vi "SRV_Sensors Variant to Data.vi"(8 "error in (no error)":errorcluster, 10 "Data":variant, 11 "Command":string) -> (0 "error out":errorcluster, 2 "Data String":string)   [LabVIEW 2014]
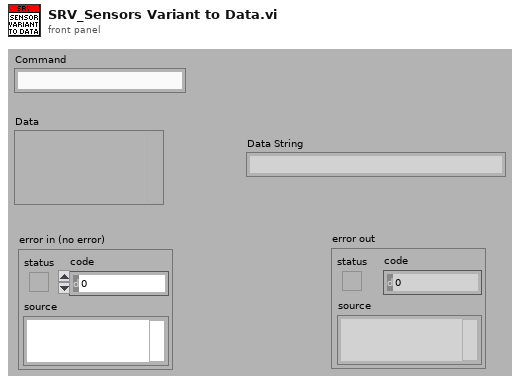
[diagram p1: front panel]
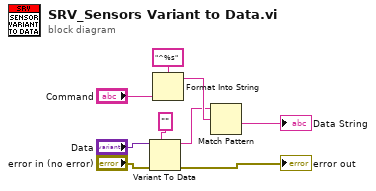
[diagram p0: block diagram]
diagram:
  n1 = Variant To Data(error in="error in (no error)", type="", Variant="Data") -> (data=w5:string, error out=→"error out":errorcluster)
  n2 = Format Into String(format string="^%s", "Command") -> (resulting string=w9:string)  [unwired: 2 in, 1 out]
  n3 = Match Pattern(string=w5, regular expression=w9) -> (after substring=→"Data String":string)  [unwired: 1 in, 3 out]
